vi "simulador.vi"(8 "error in (no error)":errorcluster, 10 "valor":dbl=0.75 format="%#_13g", 11 "CNT90.lvclass":refnum<class "CNT90.lvclass">) -> (0 "error out":errorcluster, 2 "medicion":dbl, 3 "CNT90.lvclass":refnum<class "CNT90.lvclass">)   [LabVIEW 2019, in "CNT90.lvclass"]
uses:
  CNT90.lvclass
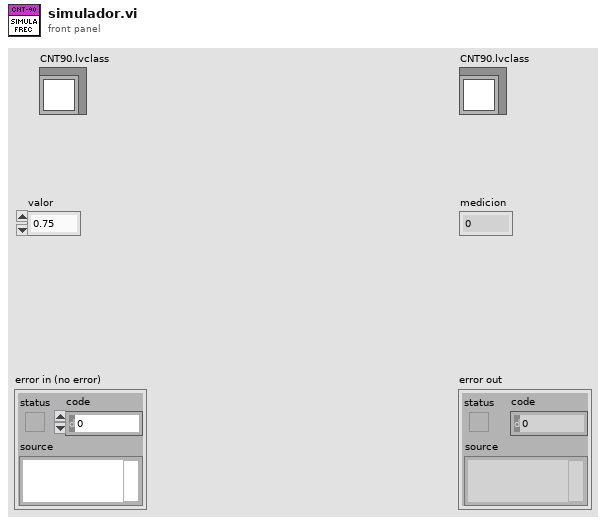
[diagram p1: front panel]
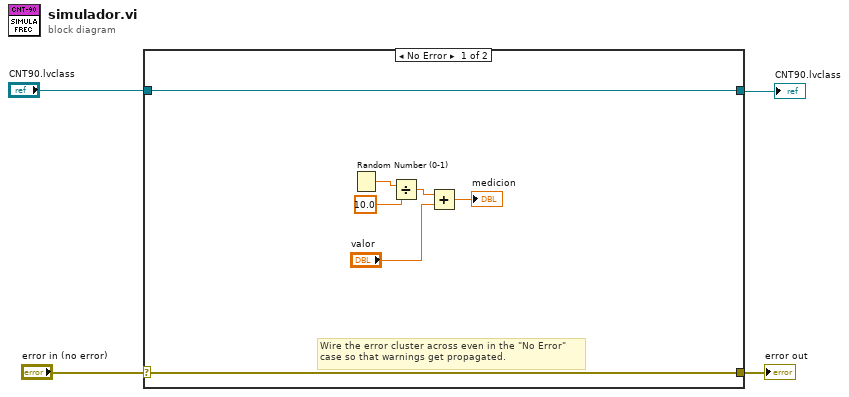
[diagram p0: block diagram]
diagram:
  n1 = case shown="No Error" "error in (no error)" {
    selector: "error in (no error)" -> [w11 w13]
    tunnel: [w11 w13] -> w3
    tunnel: [w5 w12] -> w1
    tunnel: "CNT90.lvclass" -> [w5 w12]
    frame No Error {
      # "Wire the error cluster across even in the \"No Error\"\ncase so that warnings get propagated."
      n2 = Random Number (0-1)() -> (number: 0 to 1=w9:dbl)
      n3 = Divide(x=w9, y=10.0) -> (x/y=w7:dbl)
      n4 = Add(x=w7, y="valor") -> (x+y=→"medicion":dbl)
    }
    frame Error {
    }
  }
  "error out" <- w3
  "CNT90.lvclass" <- w1
